vi "Configure Alarm Set Points.vi"(0 "VISA resource name":refnum<visa-resource-name>, 1 "Unit Address (1)":i16=1, 5 "Alarm (1)":i16=1, 7 "Alarm Low SP/Deviation (-999.0)":dbl=-999.0 format="%.2f", 9 "Alarm High SP/Deviation (999.0)":dbl=999.0 format="%.2f", 11 "error in (no error)":errorcluster {"code" format="%.0x"}) -> (4 "VISA resource name out":refnum<visa-resource-name>, 15 "error out":errorcluster {"code" format="%.0x"})   [LabVIEW 2010]
doc: "This VI configures alarm set points."
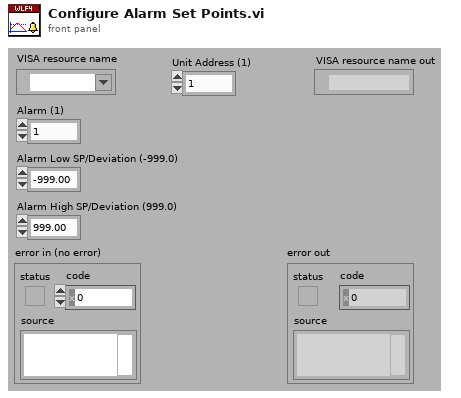
[diagram p1: front panel]
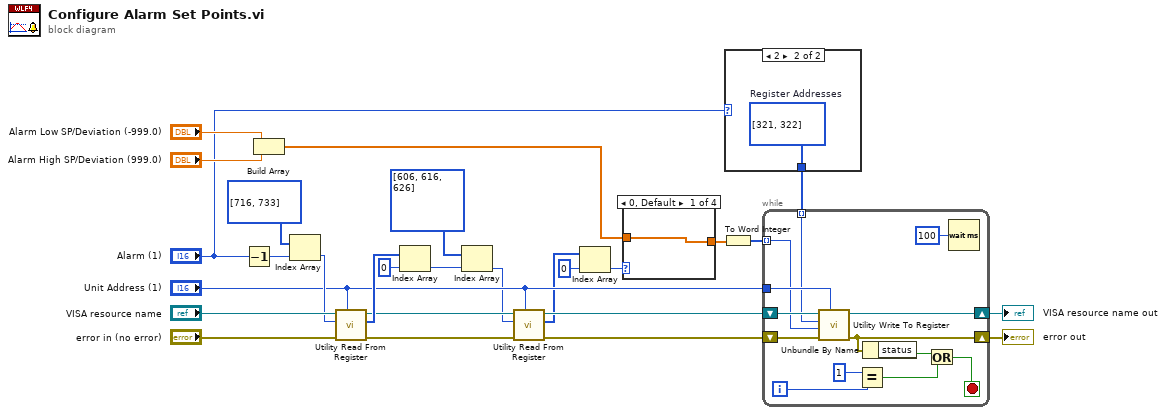
[diagram p0: block diagram]
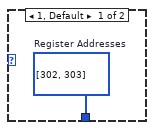
[diagram p2: hidden frame]
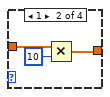
[diagram p3: hidden frame]
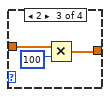
[diagram p4: hidden frame]
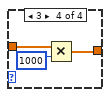
[diagram p5: hidden frame]
diagram:
  n1 = Decrement(x="Alarm (1)") -> (x-1=w22:i16)
  n2 = Build Array("Alarm Low SP/Deviation (-999.0)", "Alarm High SP/Deviation (999.0)") -> (w5:dbl[])
  n3 = Index Array(array=i32[] [716, 733], index=w22) -> (element=w21:i32)
  n4 = call "Utility Read From Register.vi"("Unit Address (1)"="Unit Address (1)", "error in (no error)"="error in (no error)", "Register Address (0)"=w21, "VISA resource name"="VISA resource name") -> ("error out"=w15:errorcluster, "Data"=w20:i16[], "VISA resource name out"=w16:refnum<visa-resource-name>)  [unwired: 5 in]
  n5 = Index Array(array=w20, index=0) -> (element=w18:i16)
  n6 = Index Array(array=i32[] [606, 616, 626], index=w18) -> (element=w11:i32)
  n7 = call "Utility Read From Register.vi"("Unit Address (1)"="Unit Address (1)", "error in (no error)"=w15, "Register Address (0)"=w11, "VISA resource name"=w16) -> ("error out"=w14:errorcluster, "Data"=w8:i16[], "VISA resource name out"=w13:refnum<visa-resource-name>)  [unwired: 5 in]
  n8 = Index Array(array=w8, index=0) -> (element=w6:i16)
  n9 = case shown="0, Default" w6 {
    tunnel: w5 -> [w28 w31 w34 w37]
    tunnel: [w28 w30 w33 w36] -> w4
    frame 0, Default {
    }
    frame 1 {
      n10 = Multiply(x=w31, y=10) -> (x*y=w30:dbl[])
    }
    frame 2 {
      n11 = Multiply(x=w34, y=100) -> (x*y=w33:dbl[])
    }
    frame 3 {
      n12 = Multiply(x=w37, y=1000) -> (x*y=w36:dbl[])
    }
  }
  n13 = To Word Integer(number=w4) -> (16bit integer=w3:i16[])
  n14 = case shown="2" "Alarm (1)" {
    tunnel: [w38 w39] -> w1
    frame 1, Default {
      w38 = i32[] [302, 303]  # Register Addresses
    }
    frame 2 {
      w39 = i32[] [321, 322]  # Register Addresses
    }
  }
  n15 = while {
    tunnel: "Unit Address (1)" -> [w52]
    shift-right: [w49] -> w27
    shift-left: w13 -> [w51]
    shift-right: [w45] -> w26
    shift-left: w14 -> [w50]
    tunnel: w1 -> [w47] mode=indexing
    tunnel: w3 -> [w46] mode=indexing
    i -> [w42]
    stop <- w43 stop-if-true
    n16 = call "Utility Write To Register.vi"("Unit Address (1)"=w52, "error in (no error)"=w50, "Data (0)"=w46, "Register Address (0)"=w47, "VISA resource name"=w51) -> ("error out"=w45:errorcluster, "VISA resource name out"=w49:refnum<visa-resource-name>)  [unwired: 5 in]
    n17 = Equal?(x=1, y=w42) -> (x = y?=w40:bool)
    n18 = Unbundle By Name(w45) -> ("status"=w44:bool)
    n19 = Or(x=w44, y=w40) -> (x .or. y?=w43:bool)
    n20 = Wait (ms)(milliseconds to wait=u32 100) -> ()  [unwired: 1 out]
  }
  "error out" <- w26
  "VISA resource name out" <- w27
